vi "Continue.vi"(9 "program":string, 10 "Telnet":refnum<k24>, 11 "error in":errorcluster) -> (0 "ErrorText":string, 1 "Succeed":bool, 2 "KclCommand":string, 3 "error out":errorcluster)   [LabVIEW 2015, in "UnderAutomation.Fanuc.lvlib"]
uses:
  UnderAutomation.Fanuc.lvlib
  C:/Users/fg/Documents/Fanuc.vi/LabVIEW_2024/UnderAutomation.Fanuc/lib/UnderAutomation.Fanuc.dll
  LabVIEW_2024/UnderAutomation.Fanuc/lib/UnderAutomation.Fanuc.dll
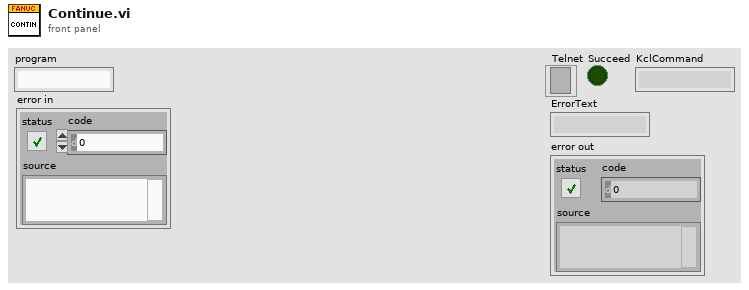
[diagram p1: front panel]
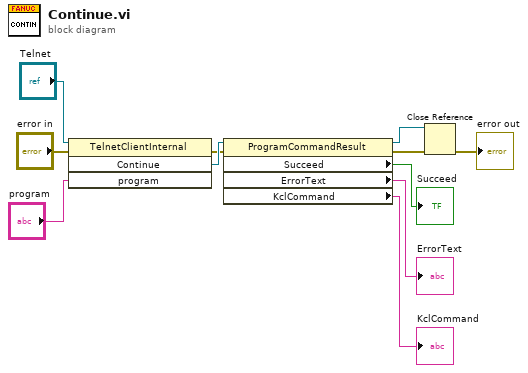
[diagram p0: block diagram]
diagram:
  n1 = invoke class="TelnetClientInternal" method="Continue"(reference="Telnet", error in="error in", "program"="program") -> (error out=w6:errorcluster, "Continue"=w9:refnum<k24>)  [unwired: 1 in, 2 out]
  n2 = property class="ProgramCommandResult"(reference=w9, error in=w6) -> (reference out=w2:refnum<k24>, error out=w3:errorcluster, "Succeed"=→"Succeed":bool, "ErrorText"=→"ErrorText":string, "KclCommand"=→"KclCommand":string)
  n3 = Close Reference(reference=w2, error in (no error)=w3) -> (error out=→"error out":errorcluster)
